vi "test14-TestArgumentInfoOfTriggeredState_State.vi"(8 "error in (no error)":errorcluster, 11 "TestCase in":refnum<class "testcase-CSMBroadcast.lvclass">) -> (0 "error out":errorcluster, 3 "TestCase out":refnum<class "testcase-CSMBroadcast.lvclass">)   [LabVIEW 2017, in "testcase-CSMBroadcast.lvclass"]
uses:
  testcase-CSMBroadcast.lvclass
  bc269a46-fbd8-4fbd-ac76-06990d02385a.vi
  8d37a2f4-20d8-4102-818c-5a8acec6f80e.vi
  src/user.lib/_NEVSTOP/Communicable State Machine(CSM)/AdvanceAPI/CSM - Get Module Attribute.vi
  <vilib>/addons/_JKI Toolkits/VI Tester/TestCase.llb/TestCase.lvclass
  src/user.lib/_NEVSTOP/Communicable State Machine(CSM)/Communicable State Machine.lvlib
  C:/Program Files (x86)/National Instruments/LabVIEW 2017/vi.lib/addons/_JKI Toolkits/VI Tester/TestCase.llb/TestCase.lvclass
panel:
  out "LoopCount":i32
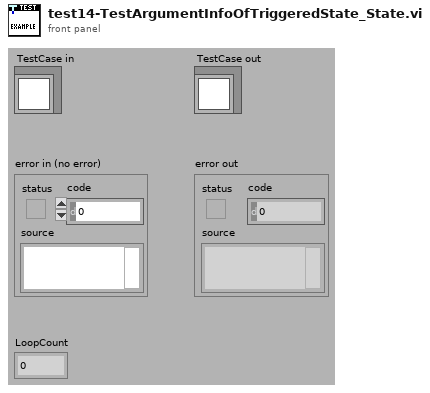
[diagram p1: front panel]
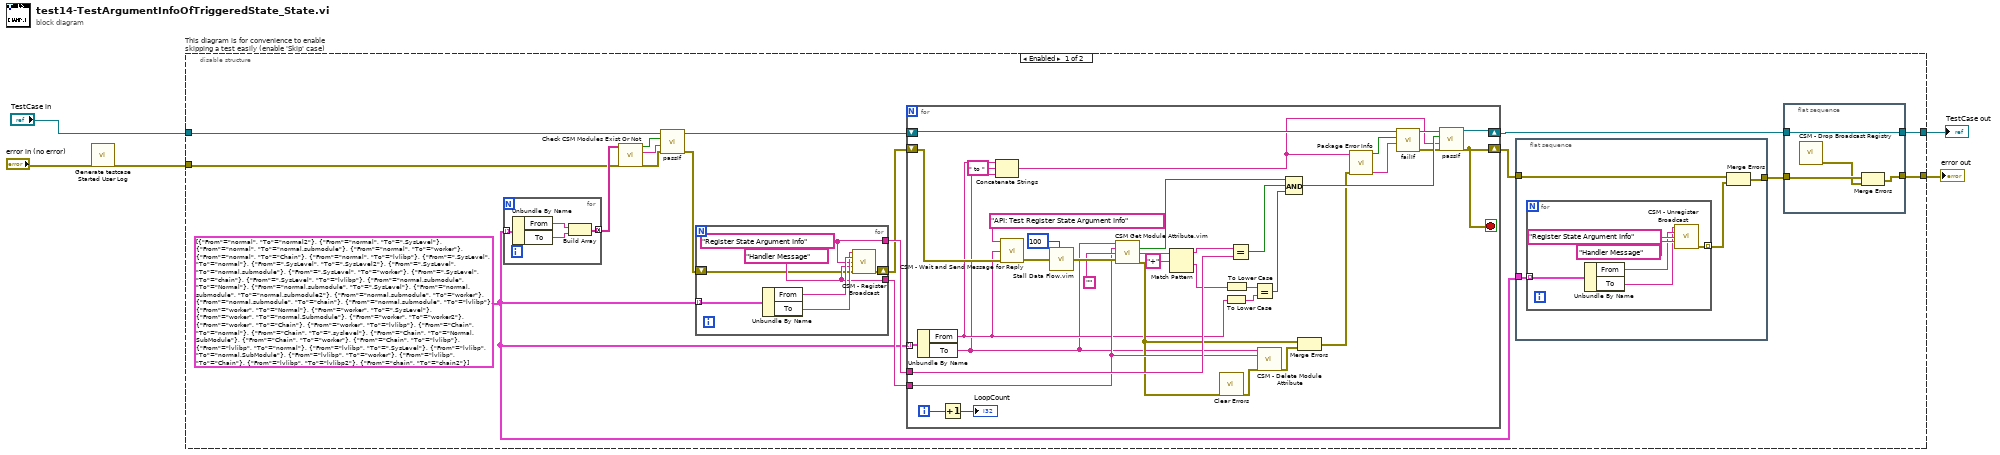
[diagram p0: block diagram]
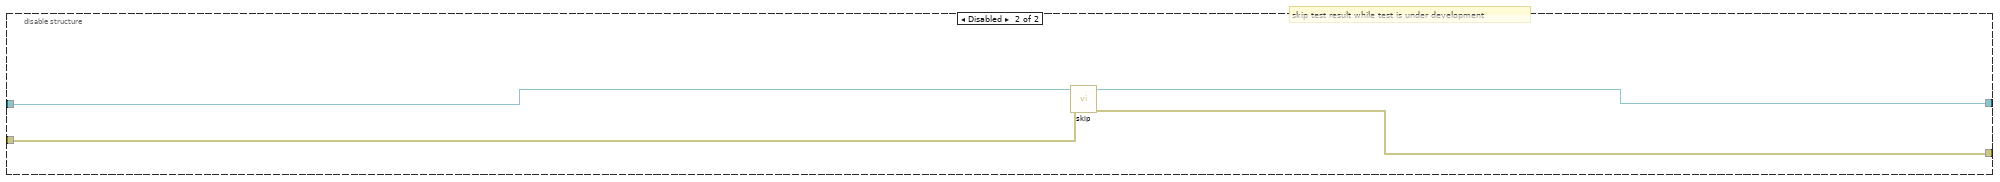
[diagram p2: hidden frame]
diagram:
  n1 = call "Generate testcase Started User Log.vi"("Error In"="error in (no error)") -> ("error out"=w1:errorcluster)  [unwired: 10 in]
  n2 = disable-structure "This diagram is for convenience to enable skipping a test easily (enable 'Skip' case)" shown="Enabled" {
    disable-tunnel: "TestCase in" -> [w10 w87]
    disable-tunnel: [w17 w85] -> w3
    disable-tunnel: [w20 w86] -> w2
    disable-tunnel: w1 -> [w9 w84]
    frame Enabled {
      w11 = cluster{"From":string, "To":string}[] [{"From"="normal", "To"="normal2"}, {"From"="normal", "To"=".SysLevel"}, {"From"="normal", "To"="normal.submodule"}, {"From"="normal", "To"="worker"}, {"From"="normal", "To"="Chain"}, {"From"="normal", "To"="lvlibp"}, {"From"=".SysLevel", "To"="normal"}, {"From"=".SysLevel", "To"=".SysLevel2"}, {"From"=".SysLevel", "To"="normal.submodule"}, {"From"=".SysLevel", "To"="worker"}, {"From"=".SysLevel", "To"="chain"}, {"From"=".SysLevel", "To"="lvlibp"}, {"From"="normal.submodule", "To"="Normal"}, {"From"="normal.submodule", "To"=".SysLevel"}, {"From"="normal.submodule", "To"="normal.submodule2"}, {"From"="normal.submodule", "To"="worker"}, {"From"="normal.submodule", "To"="chain"}, {"From"="normal.submodule", "To"="lvlibp"}, {"From"="worker", "To"="Normal"}, {"From"="worker", "To"=".SysLevel"}, {"From"="worker", "To"="normal.Submodule"}, {"From"="worker", "To"="worker2"}, {"From"="worker", "To"="Chain"}, {"From"="worker", "To"="lvlibp"}, {"From"="Chain", "To"="normal"}, {"From"="Chain", "To"=".syslevel"}, {"From"="Chain", "To"="Normal.SubModule"}, {"From"="Chain", "To"="worker"}, {"From"="Chain", "To"="lvlibp"}, {"From"="lvlibp", "To"="normal"}, {"From"="lvlibp", "To"=".SysLevel"}, {"From"="lvlibp", "To"="normal.SubModule"}, {"From"="lvlibp", "To"="worker"}, {"From"="lvlibp", "To"="Chain"}, {"From"="lvlibp", "To"="lvlibp2"}, {"From"="chain", "To"="chain2"}]
      n3 = for {
        tunnel: w11 -> [w26] mode=indexing
        tunnel: [w23] -> w14 mode=concatenating
        n4 = Unbundle By Name(w26) -> ("From"=w25:string, "To"=w24:string)
        n5 = Build Array(w25, w24) -> (w23:string[])
      }
      n6 = call "Check CSM Modules Exist Or Not.vi"("error in"=w9, "CSM names in"=w14) -> ("error out"=w12:errorcluster, "Debug string"=w13:string, "All Modules Exist?"=w15:bool)  [unwired: 7 in]
      n7 = call-dynamic "passIf.vi"("error in (no error)"=w12, "message (\"\")"=w13, "pass"=w15, "TestCase in"=w10) -> ("error out"=w7:errorcluster, "TestCase out"=w8:refnum<class "testcase-CSMBroadcast.lvclass">)  [unwired: 6 in]
      n8 = for {
        tunnel: w11 -> [w43] mode=indexing
        tunnel: [w39] -> w19
        tunnel: [w38] -> w16
        shift-right: [w40] -> w6
        shift-left: w7 -> [w37]
        w38 = "Handler Message" ("Response Message (If \"\", Same as Source Message)")
        w39 = "Register State Argument Info" ("Status")
        n9 = Unbundle By Name(w43) -> ("From"=w42:string, "To"=w41:string)
        n10 = call "CSM - Register Broadcast.vi"("CSM Name(Empty for Broadcast Event)"=w41, "Source CSM Name (* as Default)"=w42, "Trigger"=w39, "API (If \"\", Same as Trigger)"=w38, "Error In"=w37) -> ("error out"=w40:errorcluster)  [unwired: 9 in, 1 out]
      }
      n11 = for {
        tunnel: w11 -> [w82] mode=indexing
        shift-right: [w67] -> w18
        shift-left: w8 -> [w58]
        shift-right: [w65] -> w22
        shift-left: w6 -> [w55]
        tunnel: w19 -> [w73]
        tunnel: w16 -> [w64]
        i -> [w62]
        stop <- w65 stop-if-true
        n12 = Unbundle By Name(w82) -> ("From"=w51:string, "To"=w50:string)
        n13 = Increment(x=w62) -> (x+1=→"LoopCount":i32)
        n14 = Concatenate Strings(w51, " to " ("string"), w50) -> (w48:string)
        n15 = call "CSM - Wait and Send Message for Reply.vi"("State"="API: Test Register State Argument Info", "Target Module"=w51, "Error In (No Error)"=w55) -> ("error out"=w81:errorcluster)  [unwired: 9 in, 3 out]
        n16 = call "Stall Data Flow.vim"("value in"=w81, "milliseconds to wait"=u32 100) -> ("value out"=w79:errorcluster)  [unwired: 1 out]
        n17 = call "CSM Get Module Attribute.vim"("CSM Name"=w50, "Attribute"=w64, "Default Value (Empty Variant)"="", "Error In"=w79) -> ("Found"=w77:bool, "Value"=w76:string, "error out"=w54:errorcluster)  [unwired: 7 in, 2 out]
        n18 = Match Pattern(string=w76, regular expression="+") -> (before substring=w74:string, after substring=w72:string)  [unwired: 1 in, 2 out]
        n19 = call <vilib>:"Clear Errors.vi"("error in (no error)"=w54) -> ("error out"=w63:errorcluster)  [unwired: 5 in, 1 out]
        n20 = To Lower Case(string=w51) -> (all lower case string=w70:string)
        n21 = To Lower Case(string=w72) -> (all lower case string=w71:string)
        n22 = Equal?(x=w74, y=w73) -> (x = y?=w69:bool)
        n23 = Equal?(x=w71, y=w70) -> (x = y?=w68:bool)
        n24 = call "CSM - Delete Module Attribute.vi"("CSM Name"=w50, "Attribute"=w64, "Error In"=w63) -> ("error out"=w53:errorcluster)  [unwired: 9 in, 3 out]
        n25 = Compound Arithmetic op=AND(w77, w69, w68) -> (w66:bool)
        n26 = Merge Errors(w54, w53) -> (w52:errorcluster)
        n27 = call "Package Error Info.vi"("error in"=w52, "String in"=w48) -> ("packed error info out"=w59:string, "error status"=w60:bool)  [unwired: 8 in]
        n28 = call-dynamic "failIf.vi"("message (\"\")"=w59, "fail"=w60, "TestCase in"=w58) -> ("error out"=w56:errorcluster, "TestCase out"=w57:refnum<class "testcase-CSMBroadcast.lvclass">)  [unwired: 7 in]
        n29 = call-dynamic "passIf.vi"("error in (no error)"=w56, "message (\"\")"=w48, "pass"=w66, "TestCase in"=w57) -> ("error out"=w65:errorcluster, "TestCase out"=w67:refnum<class "testcase-CSMBroadcast.lvclass">)  [unwired: 6 in]
      }
      n30 = flat-sequence {
        tunnel: w11 -> [w27]
        tunnel: w22 -> [w30]
        tunnel: [w29] -> w21
        frame #0 {
          n31 = for {
            tunnel: w27 -> [w31] mode=indexing
            tunnel: [w32] -> w28 mode=indexing
            n32 = Unbundle By Name(w31) -> ("From"=w34:string, "To"=w33:string)
            n33 = call "CSM - Unregister Broadcast.vi"("CSM Name(Empty for Broadcast Event)"=w33, "Source CSM Name (* as Default)"=w34, "Trigger"="Register State Argument Info" ("Status"), "API (\"*\" as Default)"="Handler Message" ("Response Message (If \"\", Same as Source Message)")) -> ("error out"=w32:errorcluster)  [unwired: 10 in, 1 out]
          }
          n34 = Merge Errors(w30, w28) -> (w29:errorcluster)
        }
      }
      n35 = flat-sequence {
        tunnel: w21 -> [w47]
        tunnel: [w46] -> w20
        tunnel: [w45] -> w17
        tunnel: w18 -> [w45]
        frame #0 {
          n36 = call "CSM - Drop Broadcast Registry.vi"() -> ("error out"=w44:errorcluster)  [unwired: 15 in]
          n37 = Merge Errors(w47, w44) -> (w46:errorcluster)
        }
      }
    }
    frame Disabled {
      # "skip test result while test is under development"
      n38 = call <vilib>:"skip.vi"("error in (no error)"=w84, "TestCase in"=w87) -> ("error out"=w86:errorcluster, "TestCase out"=w85:refnum<class "testcase-CSMBroadcast.lvclass">)  [unwired: 8 in]
    }
  }
  "error out" <- w2
  "TestCase out" <- w3
